vi "protomodule or module.vi"(11 "assembly type":string) -> (3 "protomodule? (T)":bool)   [LabVIEW 2021]
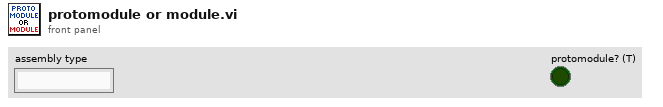
[diagram p1: front panel]
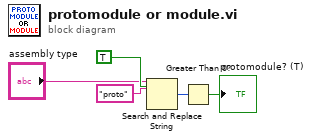
[diagram p0: block diagram]
diagram:
  n1 = Search and Replace String(case sensitive?=TRUE ("ignore case? (F)"), input string="assembly type", search string="proto") -> (number of replacements=w5:i32)  [unwired: 5 in, 3 out]
  n2 = Greater Than 0?(x=w5) -> (x > 0?=→"protomodule? (T)":bool)
